vi "Mirror Image.vi"(7 "Mirror":bool, 8 "error in (no error)":errorcluster, 10 "Symmetry":u32, 11 "Refnum in":T1) -> (0 "error out":errorcluster, 2 "Disabled":T2(ring), 3 "Refnum out":T1)   [LabVIEW 2017]
doc: "This VI flips the image in the selected symmetry."
uses:
  <vilib>/vision/Image Controls.llb/IMAQ Image.ctl
  <vilib>/vision/NI_Vision_Development_Module.lvlib
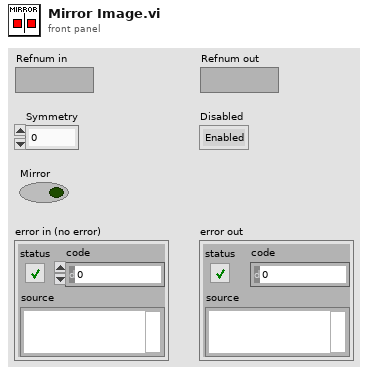
[diagram p1: front panel]
types:
  T1 = typedef "IMAQ Image.ctl" = refnum<image>
  T2 = enum8{"Enabled", "Disabled", "Disabled and Grayed Out"}
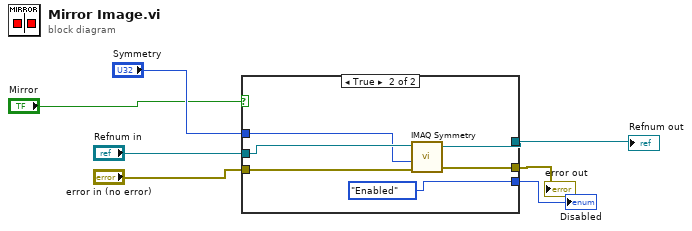
[diagram p0: block diagram]
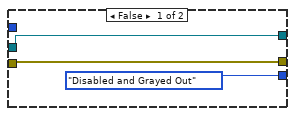
[diagram p2: hidden frame]
diagram:
  n1 = case shown="True" "Mirror" {
    tunnel: "error in (no error)" -> [w9 w12]
    tunnel: "Refnum in" -> [w10 w16]
    tunnel: [w10 w15] -> w4
    tunnel: [w9 w14] -> w6
    tunnel: "Symmetry" -> [_ w13]
    tunnel: [T2."Disabled and Grayed Out" ("Disabled") T2."Enabled" ("Disabled")] -> w7
    frame False {
    }
    frame True {
      n2 = call "IMAQ Symmetry"("error in (no error)"=w12, "Type of Symmetry"=w13, "Image Src"=w16) -> ("error out"=w14:errorcluster, "Image Dst Out"=w15:T1)  [unwired: 2 in]
    }
  }
  "Disabled" <- w7
  "error out" <- w6
  "Refnum out" <- w4
